vi "Response.vi"(0 "Response":refnum<queue>, 2 "Message (OK)":string="OK") -> ()   [LabVIEW 2014]
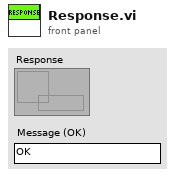
[diagram p1: front panel]
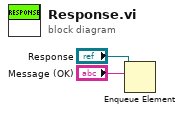
[diagram p0: block diagram]
diagram:
  n1 = Enqueue Element(queue="Response", element="Message (OK)") -> ()  [unwired: 2 in, 3 out]
